vi "Cluster Experiment.vi"() -> ()   [LabVIEW 2010]
doc: "This VI is the solution to an exercise in the LabVIEW Core I course.\n\nIt is used to enable the student to explore the cluster functions available in LabVIEW."
panel:
  out "Small Cluster":cluster{"Boolean 1":bool, "Slide value":dbl} {"Slide value" format="%.2f"}
  in  "stop":bool
  out "Boolean 2":bool
  out "Numeric":dbl format="%.2f"
  out "Modified Cluster":T1 {"Slide" scale=0.0..10.0; "Numeric" format="%.2f"}
  in  "Cluster":T1 {"Slide" scale=0.0..10.0; "Numeric" format="%.2f"}
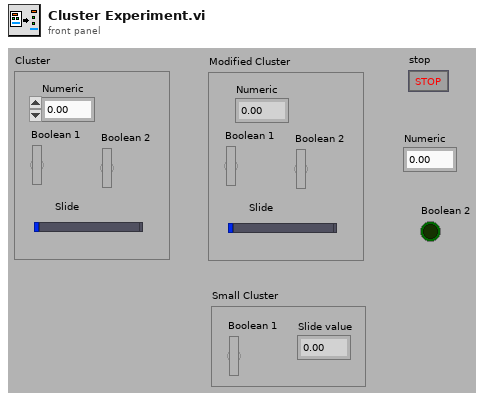
[diagram p1: front panel]
types:
  T1 = cluster{"Numeric":dbl, "Boolean 1":bool, "Boolean 2":bool, "Slide":dbl}
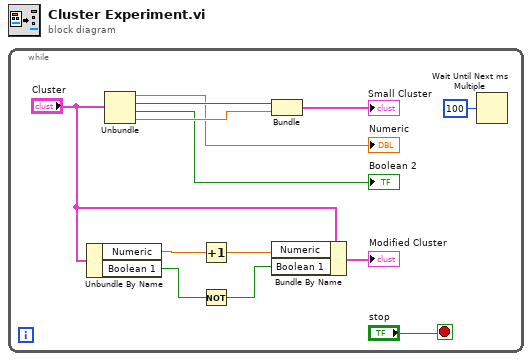
[diagram p0: block diagram]
diagram:
  n1 = while {
    stop <- "stop" stop-if-true
    n2 = Unbundle By Name "Unbundle By Name"("Cluster") -> ("Numeric"=w7:dbl, "Boolean 1"=w6:bool)
    n3 = Unbundle "Unbundle"("Cluster") -> ("Numeric"=→"Numeric":dbl, "Boolean 1"=w11:bool, "Boolean 2"=→"Boolean 2":bool, "Slide"=w12:dbl)
    n4 = Increment(x=w7) -> (x+1=w3:dbl)
    n5 = Not(x=w6) -> (.not. x?=w2:bool)
    n6 = Bundle "Bundle"("Boolean 1"=w11, "Slide"=w12) -> (→"Small Cluster":cluster{"Boolean 1":bool, "Slide":dbl})  [unwired: 1 in]
    n7 = Bundle By Name "Bundle By Name"(cluster="Cluster", "Numeric"=w3, "Boolean 1"=w2) -> (→"Modified Cluster":T1)
    n8 = Wait Until Next ms Multiple(millisecond multiple=u32 100) -> ()  [unwired: 1 out]
  }
